vi "TDMS GET DATA G2.vi"(7 "OffSet In":i32, 8 "error in":errorcluster, 10 "max":i64, 11 "tdms file In":refnum<k34>) -> (0 "error out":errorcluster, 3 "Grupo 2":T1(array[cluster]), 4 "lengh":i64, 5 "Repetir":bool)   [LabVIEW 2015]
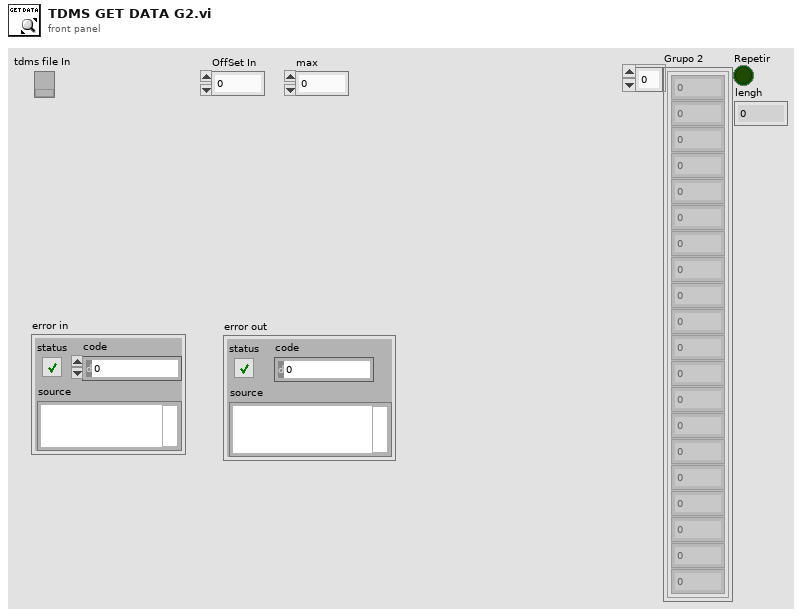
[diagram p1: front panel]
types:
  T1 = cluster{u32, dbl, dbl, dbl, dbl, dbl, dbl, dbl, dbl, dbl, dbl, dbl, dbl, dbl, dbl, dbl, dbl, dbl, dbl, dbl}[]
  T2 = cluster{u32, dbl, dbl, dbl, dbl, dbl, dbl, dbl, dbl, dbl, dbl, dbl, dbl, dbl, dbl, dbl, dbl, dbl, dbl, dbl}
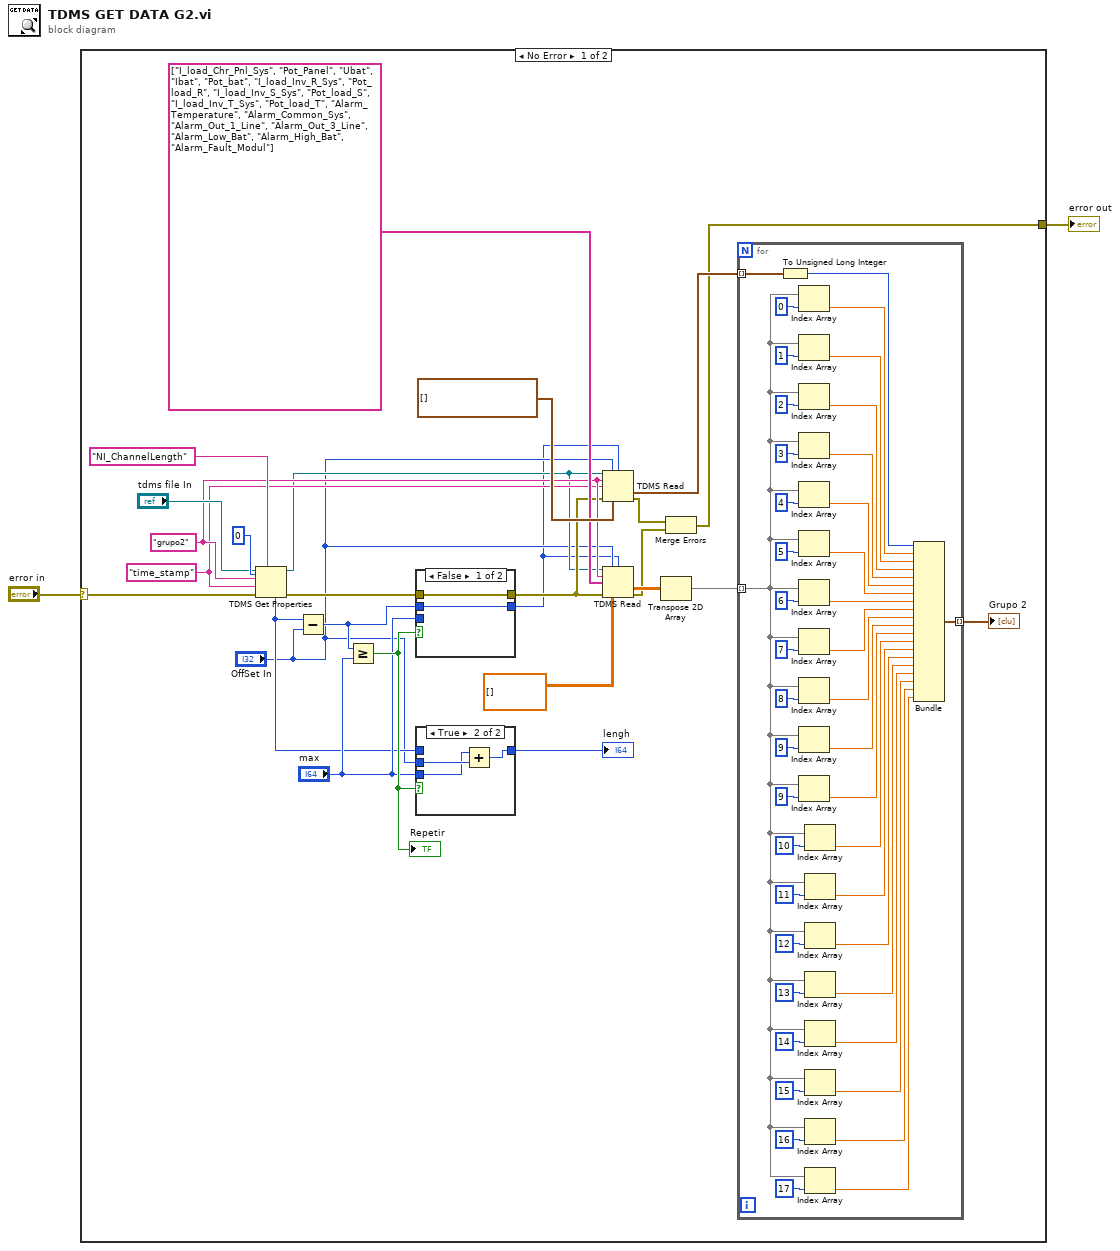
[diagram p0: block diagram]
diagram:
  n1 = case shown="No Error" "error in" {
    selector: "error in" -> [w5 w79]
    tunnel: [w4 w79] -> w1
    frame No Error {
      w12 = "time_stamp"
      w13 = "grupo2"
      n2 = TDMS Get Properties(5:0, 7:"NI_ChannelLength" ("property name"), 8:w5, 9:w12, 10:w13, 11:"tdms file In") -> (0:w10:errorcluster, 3:w8:refnum<k34>, 4:w7:i32)  [unwired: 3 out]
      n3 = Subtract(x=w7, y="OffSet In") -> (x-y=w18:i32)
      n4 = Greater Or Equal?(x=w18, y="max") -> (x >= y?=w17:bool)
      "Repetir" <- w17
      n5 = case shown="False" w17 {
        tunnel: [w34 w36] -> w3
        tunnel: w18 -> [w34 _]
        tunnel: "max" -> [_ w36]
        tunnel: w10 -> [w33 w35]
        tunnel: [w33 w35] -> w9
        frame False {
        }
        frame True {
        }
      }
      n6 = case shown="True" w17 {
        tunnel: [w29 w32] -> w16
        tunnel: w7 -> [w29 _]
        tunnel: "OffSet In" -> [_ w31]
        tunnel: "max" -> [_ w30]
        frame False {
        }
        frame True {
          n7 = Add(x=w30, y=w31) -> (x+y=w32:i64)
        }
      }
      "lengh" <- w16
      n8 = TDMS Read(0:w8, 1:"OffSet In", 2:w3, 5:w13, 7:w12, 11:w9, 12:timestamp[] []) -> (10:w26:timestamp[], 15:w14:errorcluster)  [unwired: 1 in, 4 out]
      n9 = TDMS Read(0:w8, 1:"OffSet In", 2:w3, 5:w13, 7:string[] ["I_load_Chr_Pnl_Sys", "Pot_Panel", "Ubat", "Ibat", "Pot_bat", "I_load_Inv_R_Sys", "Pot_load_R", "I_load_Inv_S_Sys", "Pot_load_S", "I_load_Inv_T_Sys", "Pot_load_T", "Alarm_Temperature", "Alarm_Common_Sys", "Alarm_Out_1_Line", "Alarm_Out_3_Line", "Alarm_Low_Bat", "Alarm_High_Bat", "Alarm_Fault_Modul"], 11:w9, 12:dbl[][] []) -> (10:w25:dbl[][], 15:w15:errorcluster)  [unwired: 1 in, 4 out]
      n10 = Transpose 2D Array(2D array=w25) -> (transposed array=w24:dbl[][])
      n11 = Merge Errors(w14, w15) -> (w4:errorcluster)
      n12 = for {
        tunnel: w26 -> [w78] mode=indexing
        tunnel: w24 -> [w40] mode=indexing
        tunnel: [w68] -> w22 mode=indexing
        n13 = To Unsigned Long Integer(number=w78) -> (unsigned 32bit integer=w73:u32)
        n14 = Index Array(array=w40, index=0) -> (element=w72:dbl)
        n15 = Index Array(array=w40, index=1) -> (element=w71:dbl)
        n16 = Index Array(array=w40, index=2) -> (element=w70:dbl)
        n17 = Index Array(array=w40, index=3) -> (element=w69:dbl)
        n18 = Index Array(array=w40, index=4) -> (element=w66:dbl)
        n19 = Index Array(array=w40, index=5) -> (element=w64:dbl)
        n20 = Index Array(array=w40, index=6) -> (element=w62:dbl)
        n21 = Index Array(array=w40, index=7) -> (element=w60:dbl)
        n22 = Index Array(array=w40, index=8) -> (element=w58:dbl)
        n23 = Index Array(array=w40, index=9) -> (element=w56:dbl)
        n24 = Index Array(array=w40, index=9) -> (element=w54:dbl)
        n25 = Index Array(array=w40, index=10) -> (element=w48:dbl)
        n26 = Index Array(array=w40, index=11) -> (element=w47:dbl)
        n27 = Index Array(array=w40, index=12) -> (element=w46:dbl)
        n28 = Index Array(array=w40, index=13) -> (element=w45:dbl)
        n29 = Index Array(array=w40, index=14) -> (element=w44:dbl)
        n30 = Index Array(array=w40, index=15) -> (element=w39:dbl)
        n31 = Index Array(array=w40, index=16) -> (element=w38:dbl)
        n32 = Index Array(array=w40, index=17) -> (element=w37:dbl)
        n33 = Bundle(w73, w72, w71, w70, w69, w66, w64, w62, w60, w58, w56, w54, w48, w47, w46, w45, w44, w39, w38, w37) -> (w68:T2)  [unwired: 1 in]
      }
      "Grupo 2" <- w22
    }
    frame Error {
    }
  }
  "error out" <- w1
